vi "Dialog - Search Sysdef for Targets.vi"(8 "error in (no error)":errorcluster, 11 "NIVS.System Definition Root":refnum<k24>) -> (0 "error out":errorcluster, 1 "Target Names":string[](array[string]), 3 "NIVS.System Defintion Root Out":refnum<k24>, 7 "Target Nodes":refnum<k24>[](array[refnum]))   [LabVIEW 2011]
uses:
  NationalInstruments.VeriStand.SystemStorage
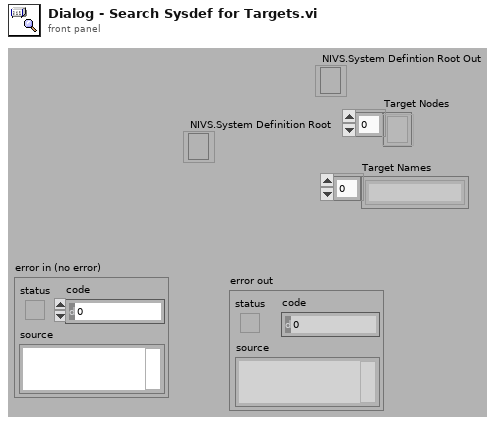
[diagram p1: front panel]
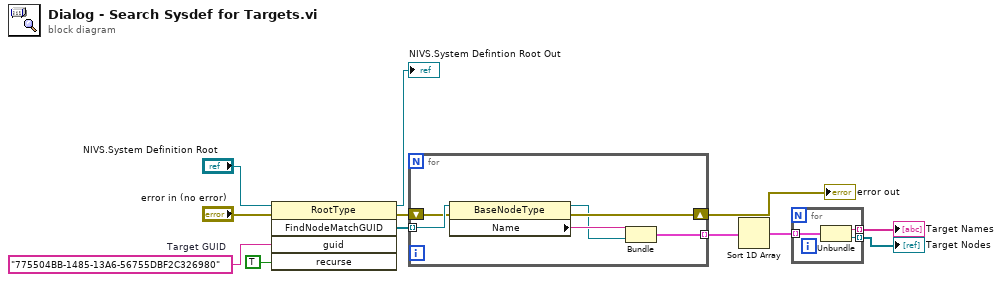
[diagram p0: block diagram]
diagram:
  w8 = "775504BB-1485-13A6-56755DBF2C326980"  # Target GUID
  n1 = invoke class="RootType" method="FindNodeMatchGUID"(reference="NIVS.System Definition Root", error in="error in (no error)", "guid"=w8, "recurse"=TRUE) -> (reference out=→"NIVS.System Defintion Root Out":refnum<k24>, error out=w6:errorcluster, "FindNodeMatchGUID"=w7:refnum<k24>[])  [unwired: 1 in, 2 out]
  n2 = for {
    tunnel: w7 -> [w18] mode=indexing
    shift-right: [w16] -> w9
    shift-left: w6 -> [w17]
    tunnel: [w13] -> w4 mode=indexing
    n3 = property class="BaseNodeType"(reference=w18, error in=w17) -> (reference out=w14:refnum<k24>, error out=w16:errorcluster, "Name"=w15:string)
    n4 = Bundle("Name"=w15, w14) -> (w13:cluster{"Name":string, refnum<k24>})  [unwired: 1 in]
  }
  "error out" <- w9
  n5 = Sort 1D Array(array=w4) -> (sorted array=w3:cluster{"Name":string, refnum<k24>}[])
  n6 = for {
    tunnel: w3 -> [w21] mode=indexing
    tunnel: [w20] -> w2 mode=indexing
    tunnel: [w19] -> w1 mode=indexing
    n7 = Unbundle(w21) -> ("Name"=w20:string, w19:refnum<k24>)
  }
  "Target Nodes" <- w1
  "Target Names" <- w2
